vi "SimpleMotion2.vi"() -> ()   [LabVIEW 2016, in "Aerotech VIs.lvlib"]
uses:
  Aerotech VIs.lvlib
  Motion/EnableMultiple.vi
  Motion/MoveIncMultiple.vi
  Motion/WaitMultiple.vi
  Motion/DisableMultiple.vi
panel:
  out "Position 2":string
  in  "Distance 2":dbl=10000.0
  in  "Speed 2":dbl=5000.0
  in  "Axis Name 2":string="Y"
  out "Position":string
  in  "Distance":dbl=10000.0
  in  "Speed":dbl=5000.0
  in  "Axis Name":string="X"
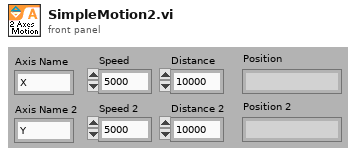
[diagram p1: front panel]
types:
  T1 = typedef "Aerotech VIs.lvlib/ControllerDiagPacket.ctl" = cluster{"Number of Diag Packets":i32, "Axes":T2[], "error":errorcluster}
  T2 = typedef "Aerotech VIs.lvlib/AxisDiagPacket.ctl" = cluster{"Axis Name":string, "Analog Input 0":dbl, "Analog Input 1":dbl, "Axis Fault (num)":i32, "Axis Fault (str)":string, "Axis Fault (bits)":cluster{"AmplifierFault":bool, "AmplifierTemperatureFault":bool, "CcwEndOfTravelLimitFault":bool, "CcwSoftwareLimitFault":bool, "CommunicationLostFault":bool, "CwEndOfTravelLimitFault":bool, "CwSoftwareLimitFault":bool, "EmergencyStopFault":bool, "EncoderFault":bool, "ExternalFault":bool, "FeedbackScalingFault":bool, "GantryMisalignFault ":bool, "HallSensorFault":bool, "InPositionTimeoutFault":bool, "MarkerSearchFault":bool, "MaxVelocityCommandFault":bool, "MotorTemperatureFault":bool, "None":bool, "OverCurrentFault":bool, "PositionErrorFault":bool, "PositionFeedbackFault":bool, "PowerSupplyFault":bool, "ProbeInputFault":bool, "SafeZoneFault":bool, "VelocityErrorFault":bool, "VelocityFeedbackFault":bool, "VoltageClampFault":bool}, "Axis Status (num)":i32, "Axis Status (str)":string, "Axis Status (bits)":cluster{"BacklashActive":bool, "CalibrationEnabled1D":bool, "CalibrationEnabled2D":bool, "CommandValid":bool, "DriveAbortPending":bool, "DrivePending":bool, "Enabling":bool, "GainMappingEnabled":bool, "GantryAligned":bool, "GantryRealigning":bool, "Homed":bool, "Homing":bool, "IFOVEnabled":bool, "JogGenerating":bool, "Jogging":bool, "JoystickControl":bool, "MasterSlaveControl":bool, "MotionBlocked":bool, "MotionClamped":bool, "MoveDone":bool, "None":bool, "NotVirtual":bool, "Profiling":bool, "Stability0":bool, "Stability1":bool, "TrajectoryFiltering":bool, "WaitDone":bool}, "Current Command":sgl, "Current Error":sgl, "Current Feedback":sgl, "Digital Inputs":i32, "Digital Outputs":i32, "Drive Status":i32, "Drive Status (str)":string, "Drive Status (bits)":cluster{"AccelerationPhase":bool, "AutofocusActive":bool, "BrakeOutput":bool, "CcwEndOfTravelLimitInput":bool, "CosineEncoderError":bool, "CurrentClamp":bool, "CwEndOfTravelLimitInput":bool, "DecelerationPhase":bool, "DualLoopActive":bool, "EmergencyStopInput":bool, "Enabled":bool, "EncoderClipping":bool, "GalvoCalibrationEnabled":bool, "GalvoPowerCorrection":bool, "HallAInput":bool, "HallBInput":bool, "HallCInput":bool, "HighResolutionMode":bool, "HomeLimitInput":bool, "InPosition":bool, "InPosition2":bool, "MarkerInput":bool, "MarkerLatch":bool, "MoveActive":bool, "NoMotorSupply":bool, "None":bool, "PowerLimiting":bool, "ProgrammingFlash":bool, "ProgrammingMXH":bool, "PSOHaltLatch":bool, "ServoControl":bool, "SineEncoderError":bool}, "Position Feedback Auxiliary":dbl, "Position Command":dbl, "Position Error":dbl, "Position Feedback":dbl, "Program Position Command":dbl, "Program Position Error":dbl, "Program Position Feedback":dbl, "Velocity Command":dbl, "Velocity Error":dbl, "Velocity Feedback":dbl}
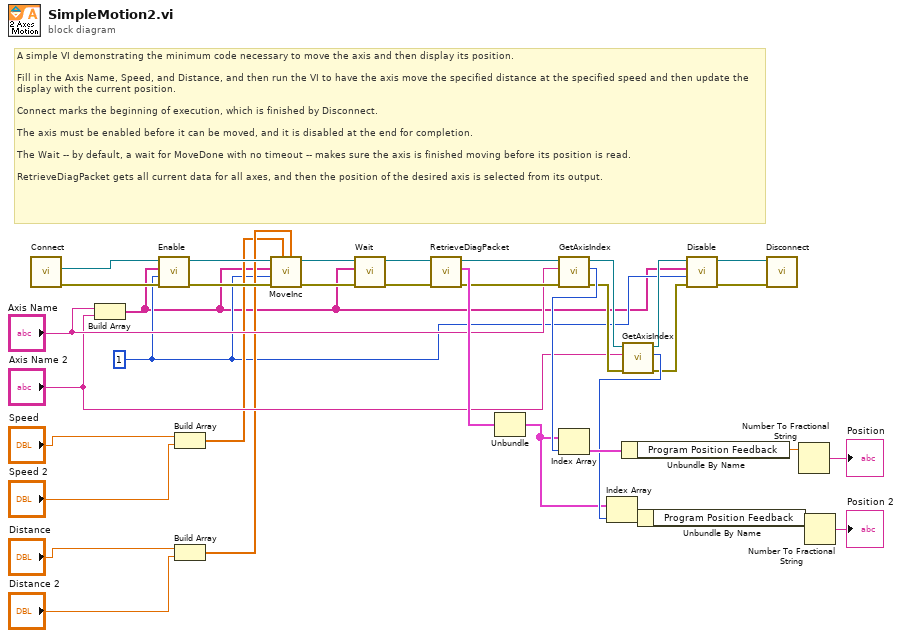
[diagram p0: block diagram]
diagram:
  w6 = 1 ("taskNumber")
  # "A simple VI demonstrating the minimum code necessary to move the axis and then display its position.\n\nFill in the Axis Name, Speed, and Distance, and then run the VI to have the axis move the specified distance at the specified speed and then update the display with the current position.\n\nConnect marks the beginning of execution, which is finished by Disconnect.\n\nThe axis must be enabled before it can be moved, and it is disabled at the end for completion.\n\nThe Wait -- by default, a wait for MoveDone with no timeout -- makes sure the axis is finished moving before its position is read.\n\nRetrieveDiagPacket gets all current data for all axes, and then the position of the desired axis is selected from its output."
  n1 = call "Connect.vi"() -> ("error out"=w16:errorcluster, "controller"=w17:refnum<k24>)  [unwired: 10 in]
  n2 = Build Array("Axis Name", "Axis Name 2") -> (w1:string[])
  n3 = call-poly "Enable.vi"("error in (no error)"=w16, "taskId"=w6, "axis names"=w1, "controller in"=w17) -> ("error out"=w15:errorcluster, "controller out"=w14:refnum<k24>)  [unwired: 6 in]
  n4 = Build Array("Speed", "Speed 2") -> (w8:dbl[])
  n5 = Build Array("Distance", "Distance 2") -> (w9:dbl[])
  n6 = call-poly "MoveInc.vi"("distances"=w9, "speeds"=w8, "error in (no error)"=w15, "taskId"=w6, "axis names"=w1, "controller in"=w14) -> ("error out"=w5:errorcluster, "controller out"=w3:refnum<k24>)  [unwired: 4 in]
  n7 = call-poly "Wait.vi"("error in (no error)"=w5, "axis names"=w1, "controller in"=w3) -> ("error out"=w4:errorcluster, "controller out"=w2:refnum<k24>)  [unwired: 6 in, 1 out]
  n8 = call "RetrieveDiagPacket.vi"("error in (no error)"=w4, "Controller In"=w2) -> ("error out"=w34:errorcluster, "ControllerDiagPacket"=w36:T1, "Controller Out"=w24:refnum<k24>)  [unwired: 7 in]
  n9 = Unbundle(w36) -> ("Axes"=w7:T2[])  [unwired: 2 out]
  n10 = call "GetAxisIndex.vi"("error in (no error)"=w34, "axis name"="Axis Name", "controller in"=w24) -> ("error out"=w25:errorcluster, "axis index"=w33:i32, "controller out"=w12:refnum<k24>)  [unwired: 6 in]
  n11 = Index Array(array=w7, index=w33) -> (element=w32:T2)
  n12 = Unbundle By Name(w32) -> ("Program Position Feedback"=w31:dbl)
  n13 = call "GetAxisIndex.vi"("error in (no error)"=w25, "axis name"="Axis Name 2", "controller in"=w12) -> ("error out"=w26:errorcluster, "axis index"=w27:i32, "controller out"=w11:refnum<k24>)  [unwired: 6 in]
  n14 = Index Array(array=w7, index=w27) -> (element=w28:T2)
  n15 = Unbundle By Name(w28) -> ("Program Position Feedback"=w30:dbl)
  n16 = call-poly "Disable.vi"("error in (no error)"=w26, "taskId"=w6, "axis names"=w1, "controller in"=w11) -> ("error out"=w13:errorcluster, "controller out"=w10:refnum<k24>)  [unwired: 6 in]
  n17 = call "Disconnect.vi"("error in (no error)"=w13, "controller"=w10) -> ()  [unwired: 9 in, 1 out]
  n18 = Number To Fractional String(number=w31) -> (F-format string=→"Position":string)  [unwired: 3 in]
  n19 = Number To Fractional String(number=w30) -> (F-format string=→"Position 2":string)  [unwired: 3 in]
